vi "Create SmtpClient.vi"(7 "host":string, 8 "error in (no error)":errorcluster caption="错误输入（无错误）", 9 "password":string, 10 "userName":string, 11 "Email In":refnum<class "Email.lvclass"> caption="DNL_LabVIEW Object in") -> (0 "error out":errorcluster caption="错误输出", 3 "Email Out":refnum<class "Email.lvclass"> caption="DNL_LabVIEW Object out")   [LabVIEW 2012, in "Email.lvclass"]
uses:
  Email.lvclass
  Email.lvclass/Email.ctl
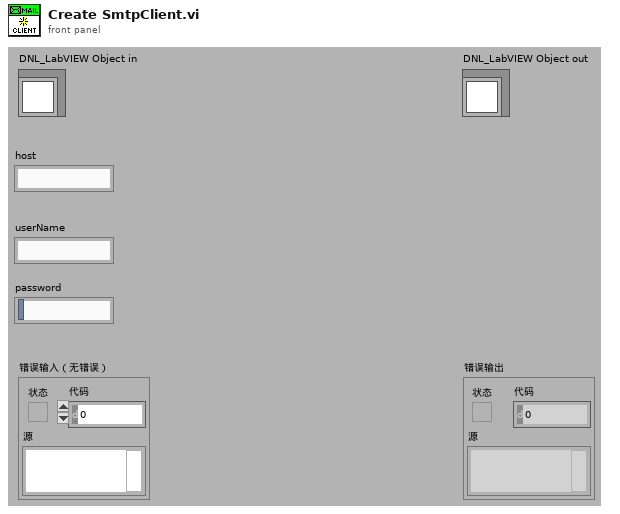
[diagram p1: front panel]
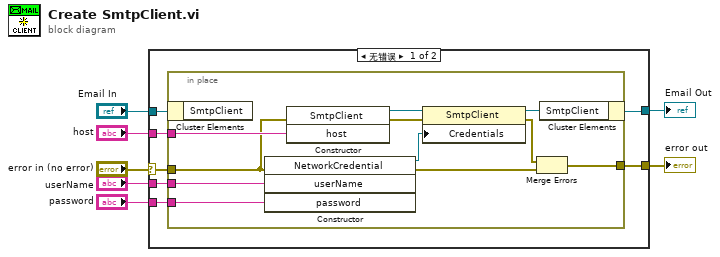
[diagram p0: block diagram]
diagram:
  n1 = case shown="无错误" "error in (no error)" {
    selector: "error in (no error)" -> [w10 w27]
    tunnel: [w9 w27] -> w6
    tunnel: [w8 w26] -> w4
    tunnel: "Email In" -> [w14 w26]
    tunnel: "host" -> [w13 _]
    tunnel: "password" -> [w12 _]
    tunnel: "userName" -> [w11 _]
    frame No Error {
      n2 = in-place {
        in-place-border: w13 -> [w25]
        in-place-border: w12 -> [w24]
        in-place-border: w11 -> [w23]
        in-place-border: w10 -> [w18]
        in-place-border: [w15] -> w9
        n3 = in-place-cluster #1(w14) -> ()  [unwired: 1 out]
        n4 = constructor class="NetworkCredential"(error in=w18, "userName"=w23, "password"=w24) -> (reference out=w21:refnum<k24>, error out=w16:errorcluster)  [unwired: 2 in, 3 out]
        n5 = constructor class="SmtpClient"(error in=w18, "host"=w25) -> (reference out=w20:refnum<k24>, error out=w22:errorcluster)  [unwired: 2 in, 2 out]
        n6 = property class="SmtpClient"(reference=w20, error in=w22, "Credentials"=w21) -> (reference out=w19:refnum<k24>, error out=w17:errorcluster)
        n7 = Merge Errors(w17, w16) -> (w15:errorcluster)
        n8 = in-place-cluster #1("SmtpClient"=w19) -> (w8:refnum<class "Email.lvclass">)
      }
    }
    frame Error {
    }
  }
  "error out" <- w6
  "Email Out" <- w4
